vi "FVIR_LDO_Oil_Machine.vi"(8 "error in":errorcluster, 11 "Message Queues":T1) -> (0 "error out":errorcluster)   [LabVIEW 2020]
uses:
  Message Queue/All Message Queues.ctl
  Message Queue/Message Cluster.ctl
  Drivers/Unist Quantum/Type Definitions/UNIST Fluid Rate.ctl
  Message Queue/Enqueue Message (Single).vi
  Message Queue/Message Queue.lvlib
panel:
  out "Numeric":i32
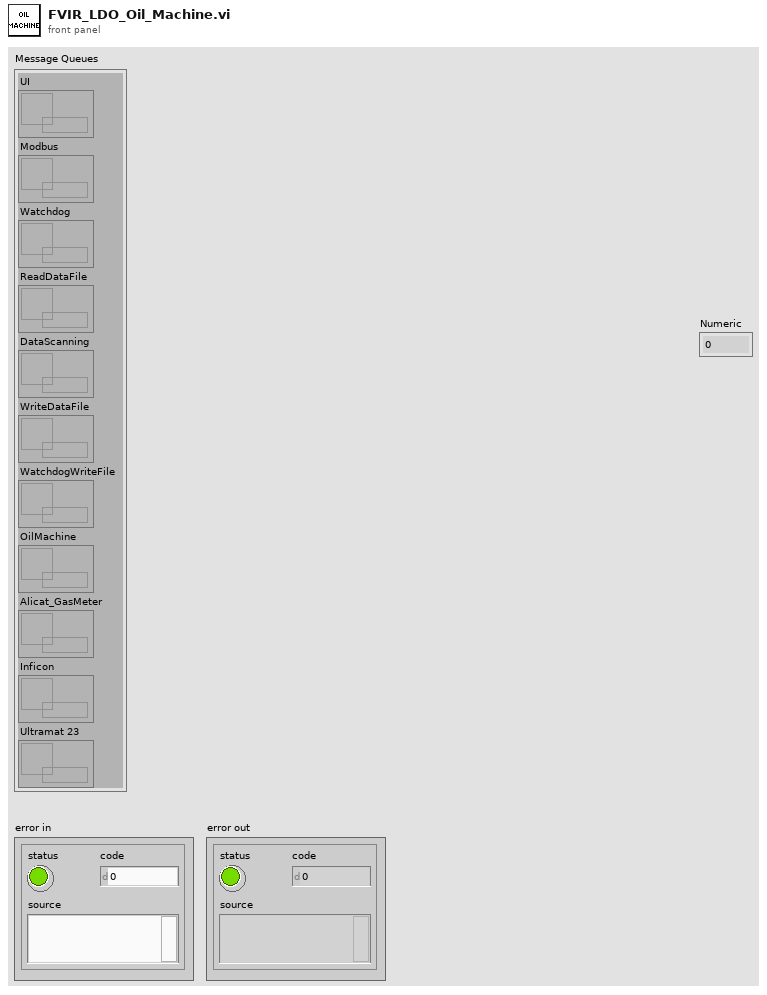
[diagram p1: front panel]
types:
  T1 = typedef "Message Queue.lvlib/All Message Queues.ctl" = cluster{"UI":refnum<queue>, "Modbus":refnum<queue>, "Watchdog":refnum<queue>, "ReadDataFile":refnum<queue>, "DataScanning":refnum<queue>, "WriteDataFile":refnum<queue>, "WatchdogWriteFile":refnum<queue>, "OilMachine":refnum<queue>, "Alicat_GasMeter":refnum<queue>, "Inficon":refnum<queue>, "Ultramat 23":refnum<queue>}
  T2 = typedef "UNIST Fluid Rate.ctl" = string
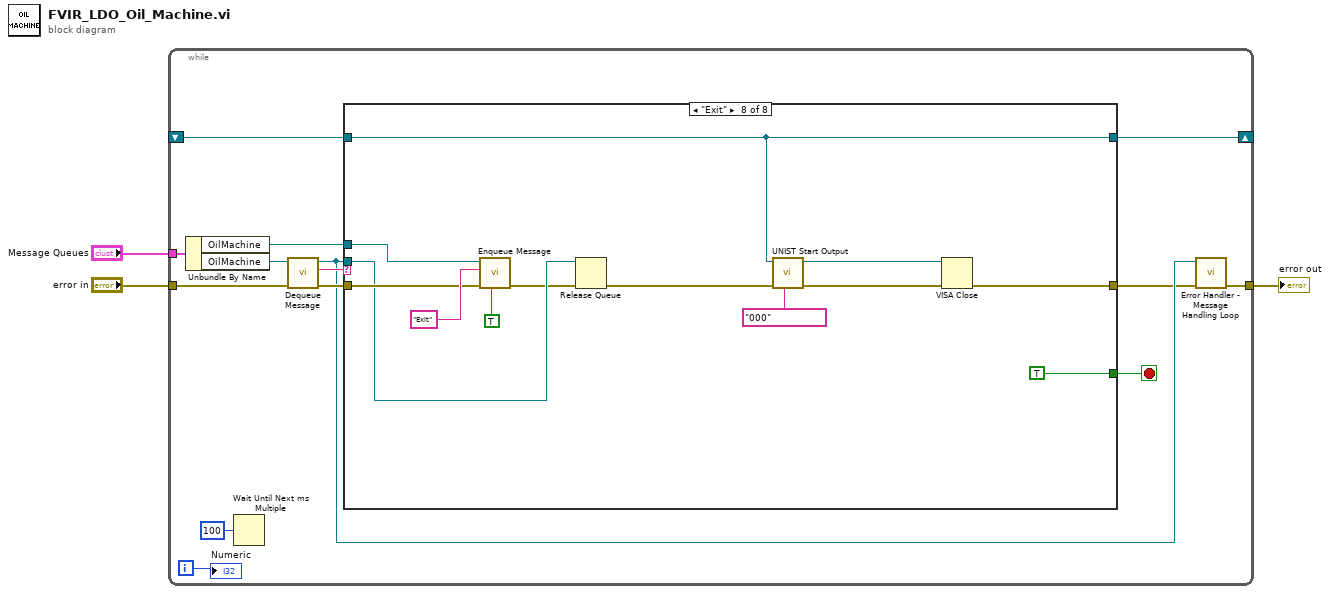
[diagram p0: block diagram]
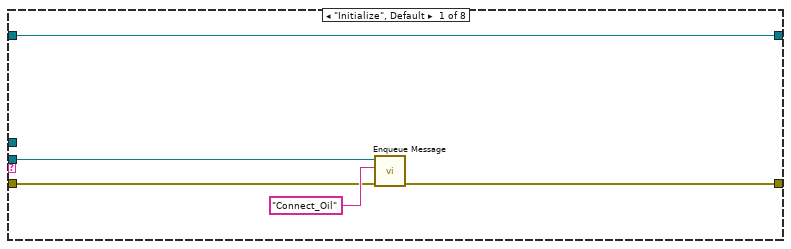
[diagram p2: hidden frame]
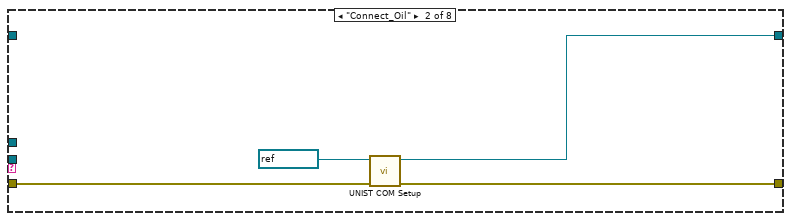
[diagram p3: hidden frame]
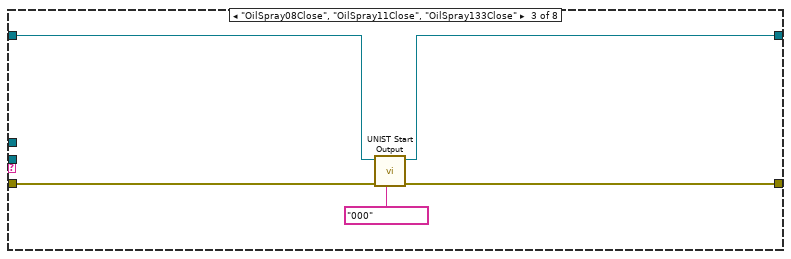
[diagram p4: hidden frame]
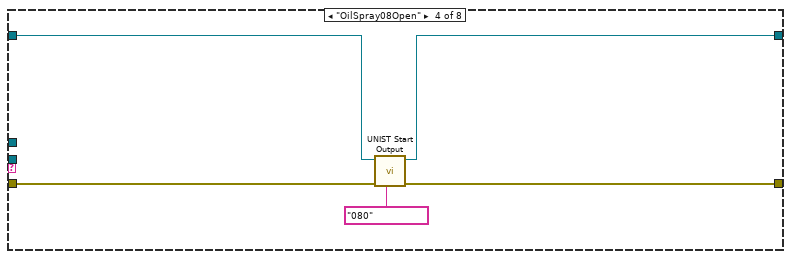
[diagram p5: hidden frame]
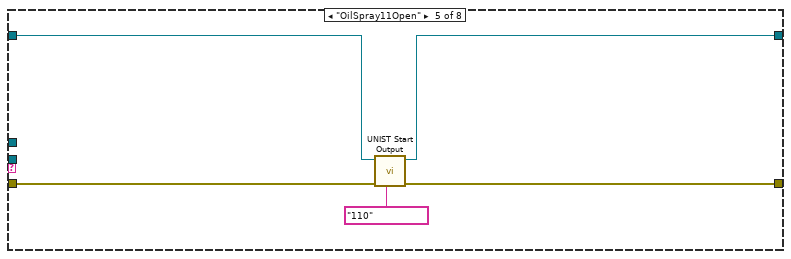
[diagram p6: hidden frame]
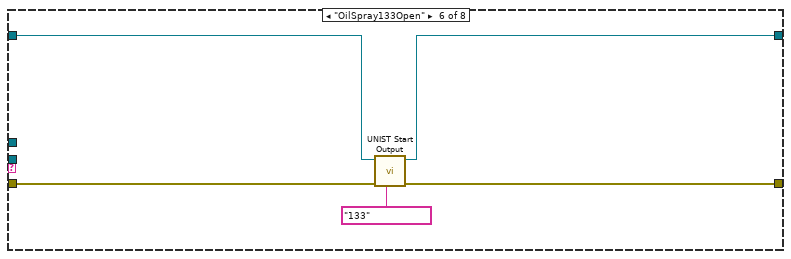
[diagram p7: hidden frame]
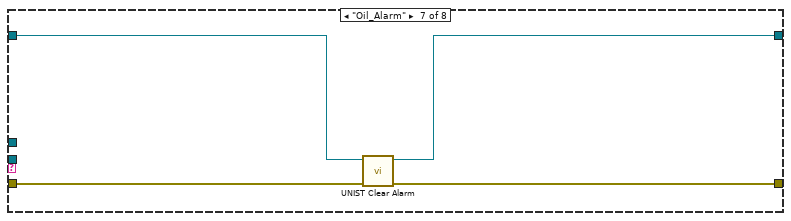
[diagram p8: hidden frame]
diagram:
  n1 = while {
    tunnel: "Message Queues" -> [w17]
    tunnel: "error in" -> [w15]
    tunnel: [w9] -> w1
    shift-right: [w7] -> _
    shift-left: _ -> [w6]
    i -> [w4]
    stop <- w12 stop-if-true
    n2 = Unbundle By Name(w17) -> ("OilMachine"=w11:refnum<queue>, "OilMachine"=w16:refnum<queue>)
    n3 = Wait Until Next ms Multiple(millisecond multiple=u32 100) -> ()  [unwired: 1 out]
    n4 = call "Dequeue Message.vi"("error in (no error)"=w15, "Message Queue"=w16) -> ("error out"=w13:errorcluster, "Message"=w14:string, "dup Message Queue"=w10:refnum<queue>)  [unwired: 6 in, 1 out]
    n5 = case shown="\"Exit\"" w14 {
      tunnel: w13 -> [w20 w26 w31 w36 w41 w46 w50 w59]
      tunnel: [w19 w25 w30 w35 w40 w45 w49 w56] -> w8
      tunnel: [_ _ _ _ _ _ _ TRUE] -> w12
      tunnel: w11 -> [_ _ _ _ _ _ _ w60]
      tunnel: w10 -> [w18 _ _ _ _ _ _ w58]
      tunnel: [w22 w23 w28 w33 w38 w43 w47 w52] -> w7
      tunnel: w6 -> [w22 _ w29 w34 w39 w44 w48 w52]
      frame "Initialize", Default {
        n6 = call-poly "Enqueue Message.vi"("error in (no error)"=w20, "Message"="Connect_Oil", "Message Queue"=w18) -> ("error out"=w19:errorcluster)  [unwired: 7 in, 1 out]
      }
      frame "Connect_Oil" {
        n7 = call "UNIST COM Setup.vi"("error in (no error)"=w26, "VISA Refnum in"=refnum<visa-resource-name> "UNIST") -> ("error out"=w25:errorcluster, "VISA Refnum out"=w23:refnum<visa-resource-name>)  [unwired: 8 in]
      }
      frame "OilSpray08Close", "OilSpray11Close", "OilSpray133Close" {
        n8 = call "UNIST Start Output.vi"("Fluid Rate (CC/MIN)"=T2 "000", "error in (no error)"=w31, "VISA Refnum in"=w29) -> ("error out"=w30:errorcluster, "VISA Refnum out"=w28:refnum<visa-resource-name>)  [unwired: 7 in]
      }
      frame "OilSpray08Open" {
        n9 = call "UNIST Start Output.vi"("Fluid Rate (CC/MIN)"=T2 "080", "error in (no error)"=w36, "VISA Refnum in"=w34) -> ("error out"=w35:errorcluster, "VISA Refnum out"=w33:refnum<visa-resource-name>)  [unwired: 7 in]
      }
      frame "OilSpray11Open" {
        n10 = call "UNIST Start Output.vi"("Fluid Rate (CC/MIN)"=T2 "110", "error in (no error)"=w41, "VISA Refnum in"=w39) -> ("error out"=w40:errorcluster, "VISA Refnum out"=w38:refnum<visa-resource-name>)  [unwired: 7 in]
      }
      frame "OilSpray133Open" {
        n11 = call "UNIST Start Output.vi"("Fluid Rate (CC/MIN)"=T2 "133", "error in (no error)"=w46, "VISA Refnum in"=w44) -> ("error out"=w45:errorcluster, "VISA Refnum out"=w43:refnum<visa-resource-name>)  [unwired: 7 in]
      }
      frame "Oil_Alarm" {
        n12 = call "UNIST Clear Alarm.vi"("error in (no error)"=w50, "VISA Refnum in"=w48) -> ("error out"=w49:errorcluster, "VISA Refnum out"=w47:refnum<visa-resource-name>)  [unwired: 8 in]
      }
      frame "Exit" {
        n13 = call-poly "Enqueue Message.vi"("Priority Message? (F)"=TRUE, "error in (no error)"=w59, "Message"="Exit", "Message Queue"=w60) -> ("error out"=w57:errorcluster)  [unwired: 6 in, 1 out]
        n14 = Release Queue(queue=w58, error in (no error)=w57) -> (error out=w54:errorcluster)  [unwired: 1 in, 2 out]
        n15 = call "UNIST Start Output.vi"("Fluid Rate (CC/MIN)"=T2 "000", "error in (no error)"=w54, "VISA Refnum in"=w52) -> ("error out"=w53:errorcluster, "VISA Refnum out"=w51:refnum<visa-resource-name>)  [unwired: 7 in]
        n16 = VISA Close(VISA resource name=w51, error in (no error)=w53) -> (error out=w56:errorcluster)
      }
    }
    n17 = call "Error Handler - Message Handling Loop.vi"("error in (no error)"=w8, "Message Queue"=w10) -> ("dup error in"=w9:errorcluster)  [unwired: 8 in, 1 out]
    "Numeric" <- w4
  }
  "error out" <- w1
